vi "Teleop.vi"(9 "Match Info":T1={"Autonomous Elapsed Seconds"=0.0, "TeleOp Elapsed Seconds"=0.0, "Disabled Elapsed Seconds"=0.0, "Visited Autonomous"=FALSE, "Visited TeleOp"=FALSE, "Visited Disabled"=FALSE, "Autonomous Settings"={"Autonomous Style"=enum."Independent", "VI Refnum"=refnum}}, 11 "Call Context":T2) -> ()   [LabVIEW 2017]
doc: "This VI is called for each TeleOp packet received from the DS where the robot is not disabled. It is often used to read from the joysticks and update I/O or to update setpoints for timed control loops. It should complete and return within 20 milliseconds or it may miss DS packets."
uses:
  <vilib>/Rock Robotics/WPI/DriverStation/WPI_DriverStationDerivedRobotMode.ctl
  <vilib>/Rock Robotics/WPI/DriverStation/WPI_DriverStationMatch Info.ctl
  <vilib>/Rock Robotics/WPI/Utilities/WPI_GetSetVariantRefNum.vi
  <vilib>/Rock Robotics/Network Tables/NT Write Boolean.vi
  <vilib>/Rock Robotics/Network Tables/NT Read Boolean.vi
  <vilib>/Rock Robotics/Network Tables/NT Read Number.vi
panel:
  out "Sample Slider 0":dbl(slide) scale=0.0..5.0
  out "Sample Boolean 1":bool
  out "Sample Boolean 0":bool
  # "what we want"
  # "actual"
  # "0.005740418607"
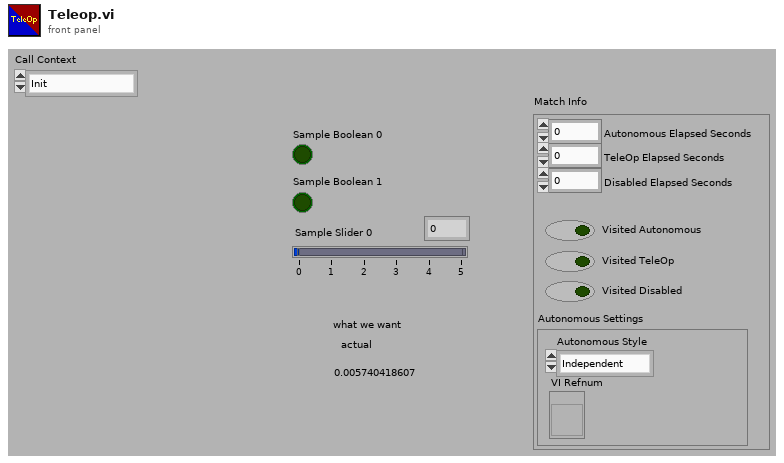
[diagram p1: front panel]
types:
  T1 = typedef "WPI_DriverStationMatch Info.ctl" = cluster{"Autonomous Elapsed Seconds":dbl, "TeleOp Elapsed Seconds":dbl, "Disabled Elapsed Seconds":dbl, "Visited Autonomous":bool, "Visited TeleOp":bool, "Visited Disabled":bool, "Autonomous Settings":cluster{"Autonomous Style":enum16{"Iterative", "Independent"}, "VI Refnum":refnum<vi>}}
  T2 = typedef "WPI_DriverStationDerivedRobotMode.ctl" = enum16{"Init", "Execute", "Stop"}
  T3 = typedef "WPI_JoystickDevRef.ctl" = cluster{"Device":T4}
  T4 = typedef "WPI_JoystickDeviceEnum.ctl" = enum16{"USB 0", "USB 1", "USB 2", "USB 3", "USB 4", "USB 5"}
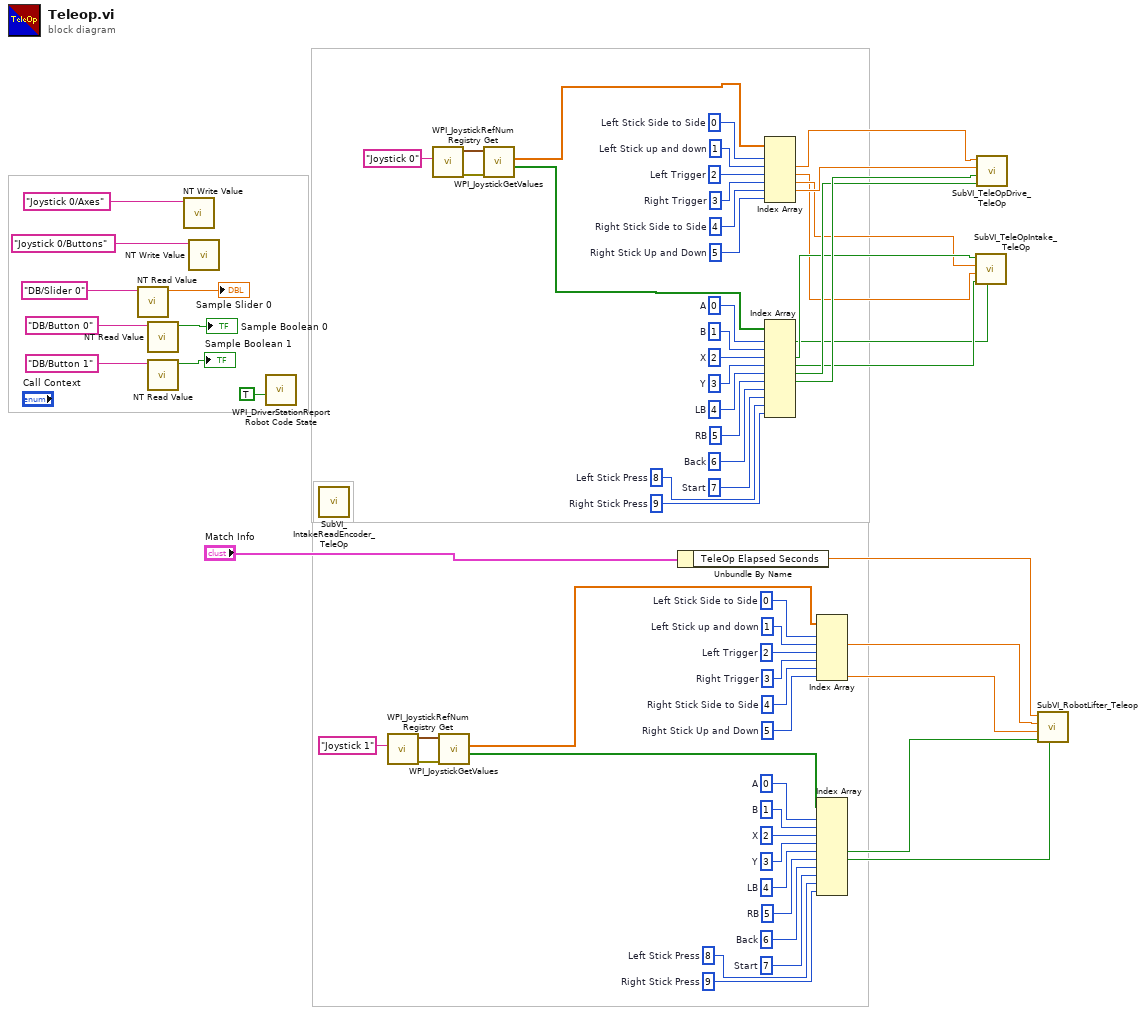
[diagram p0: block diagram]
diagram:
  w18 = 5  # Right Stick Up and Down
  w19 = 4  # Right Stick Side to Side
  w20 = 3  # Right Trigger
  w21 = 2  # Left Trigger
  w22 = 1  # Left Stick up and down
  w23 = 0  # Left Stick Side to Side
  w24 = 9  # Right Stick Press
  w25 = 8  # Left Stick Press
  w26 = 7  # Start
  w27 = 6  # Back
  w28 = 5  # RB
  w29 = 4  # LB
  w30 = 3  # Y
  w31 = 2  # X
  w32 = 1  # B
  w33 = 0  # A
  w36 = 5  # Right Stick Up and Down
  w37 = 4  # Right Stick Side to Side
  w38 = 3  # Right Trigger
  w39 = 2  # Left Trigger
  w40 = 1  # Left Stick up and down
  w41 = 0  # Left Stick Side to Side
  w42 = 9  # Right Stick Press
  w43 = 8  # Left Stick Press
  w44 = 7  # Start
  w45 = 6  # Back
  w46 = 5  # RB
  w47 = 4  # LB
  w48 = 3  # Y
  w49 = 2  # X
  w50 = 1  # B
  w51 = 0  # A
  n1 = call-poly <vilib>:"NT Read Value.vi"("Name"="DB/Slider 0" ("refnum name")) -> ("Numeric"=→"Sample Slider 0":dbl)  [unwired: 9 in, 1 out]
  n2 = call-poly <vilib>:"NT Read Value.vi"("Name"="DB/Button 0" ("refnum name")) -> ("Boolean"=→"Sample Boolean 0":bool)  [unwired: 9 in, 1 out]
  n3 = call-poly <vilib>:"NT Read Value.vi"("Name"="DB/Button 1" ("refnum name")) -> ("Boolean"=→"Sample Boolean 1":bool)  [unwired: 9 in, 1 out]
  n4 = call-poly <vilib>:"NT Write Value.vi"("Name"="Joystick 0/Axes") -> ()  [unwired: 10 in, 1 out]
  n5 = call-poly <vilib>:"NT Write Value.vi"("Name"="Joystick 0/Buttons") -> ()  [unwired: 10 in, 1 out]
  n6 = call <vilib>:"WPI_DriverStationReport Robot Code State.vi"("TeleOp"=TRUE ("Autonomous")) -> ()  [unwired: 10 in, 1 out]
  n7 = call "SubVI_IntakeReadEncoder_TeleOp.vi"() -> ()  [unwired: 12 in]
  n8 = call <vilib>:"WPI_JoystickRefNum Registry Get.vi"("refnum name"="Joystick 1") -> ("error out"=w54:errorcluster, "JoystickDevRef"=w52:T3)  [unwired: 1 in, 8 out]
  n9 = call <vilib>:"WPI_JoystickRefNum Registry Get.vi"("refnum name"="Joystick 0") -> ("error out"=w55:errorcluster, "JoystickDevRef"=w64:T3)  [unwired: 1 in, 8 out]
  n10 = call <vilib>:"WPI_JoystickGetValues.vi"("error in (no error)"=w54, "JoystickDevRef"=w52) -> ("Buttons"=w16:bool[], "Axes"=w17:dbl[])  [unwired: 5 in, 3 out]
  n11 = call <vilib>:"WPI_JoystickGetValues.vi"("error in (no error)"=w55, "JoystickDevRef"=w64) -> ("Buttons"=w34:bool[], "Axes"=w35:dbl[])  [unwired: 5 in, 3 out]
  n12 = Unbundle By Name("Match Info") -> ("TeleOp Elapsed Seconds"=w14:dbl)
  n13 = Index Array(array=w35, index #1=w41, index #2=w40, index #3=w39, index #4=w38, index #5=w37, index #6=w36) -> (element #2=w1:dbl, element #3=w8:dbl, element #4=w9:dbl, element #5=w13:dbl)  [unwired: 2 out]
  n14 = Index Array(array=w34, index #1=w51, index #2=w50, index #3=w49, index #4=w48, index #5=w47, index #6=w46, index #7=w45, index #8=w44, index #9=w43, index #10=w42) -> (element #1=w3:bool, element #3=w10:bool, element #4=w4:bool, element #5=w11:bool, element #6=w12:bool)  [unwired: 5 out]
  n15 = Index Array(array=w17, index #1=w23, index #2=w22, index #3=w21, index #4=w20, index #5=w19, index #6=w18) -> (element #2=w6:dbl, element #6=w5:dbl)  [unwired: 4 out]
  n16 = Index Array(array=w16, index #1=w33, index #2=w32, index #3=w31, index #4=w30, index #5=w29, index #6=w28, index #7=w27, index #8=w26, index #9=w25, index #10=w24) -> (element #5=w7:bool, element #6=w2:bool)  [unwired: 8 out]
  n17 = call "SubVI_TeleOpIntake_TeleOp.vi"("Open/close Intake"=w3, "SpitCube"=w4, 9:"placeholder intake lift"=w8, 10:"placeholder intake lift"=w9, "TakeInCube"=w10) -> ()  [unwired: 7 in]
  n18 = call "SubVI_TeleOpDrive_TeleOp.vi"("DriveShiftLow"=w11, "DriveShiftHigh"=w12, "X axis"=w13, "Y axis"=w1) -> ()  [unwired: 8 in]
  n19 = call "SubVI_RobotLifter_Teleop.vi"("(Button)LifterReset"=w2, "(Button)LifterDeploy"=w7, "RightClimber"=w5, "LeftClimber"=w6, "TeleOp Elapsed Seconds"=w14) -> ()  [unwired: 6 in, 1 out]
